vi "VI malcriado.vi"(8 "error in":errorcluster, 11 "This VI":refnum<vi>) -> ()   [LabVIEW 2024]
uses:
  <vilib>/Utility/miscctls.llb/LVRowAndColumnTypeDef.ctl
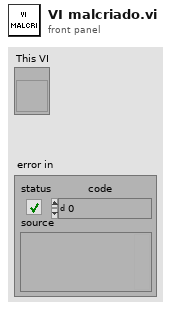
[diagram p1: front panel]
types:
  T1 = typedef "Pdash Style--cluster.ctl" = cluster{"Gris Obscuro Azul":u32, "Gris Medio Azul":u32, "Gris Claro Azul":u32, "Amarillo":u32, "Text color":u32, "Transparent":u32, "Fuente":string, "Text.Font:Size":u32}
  T2 = typedef "LVRowAndColumnTypeDef.ctl" = cluster{"Row":i32, "Column":i32}
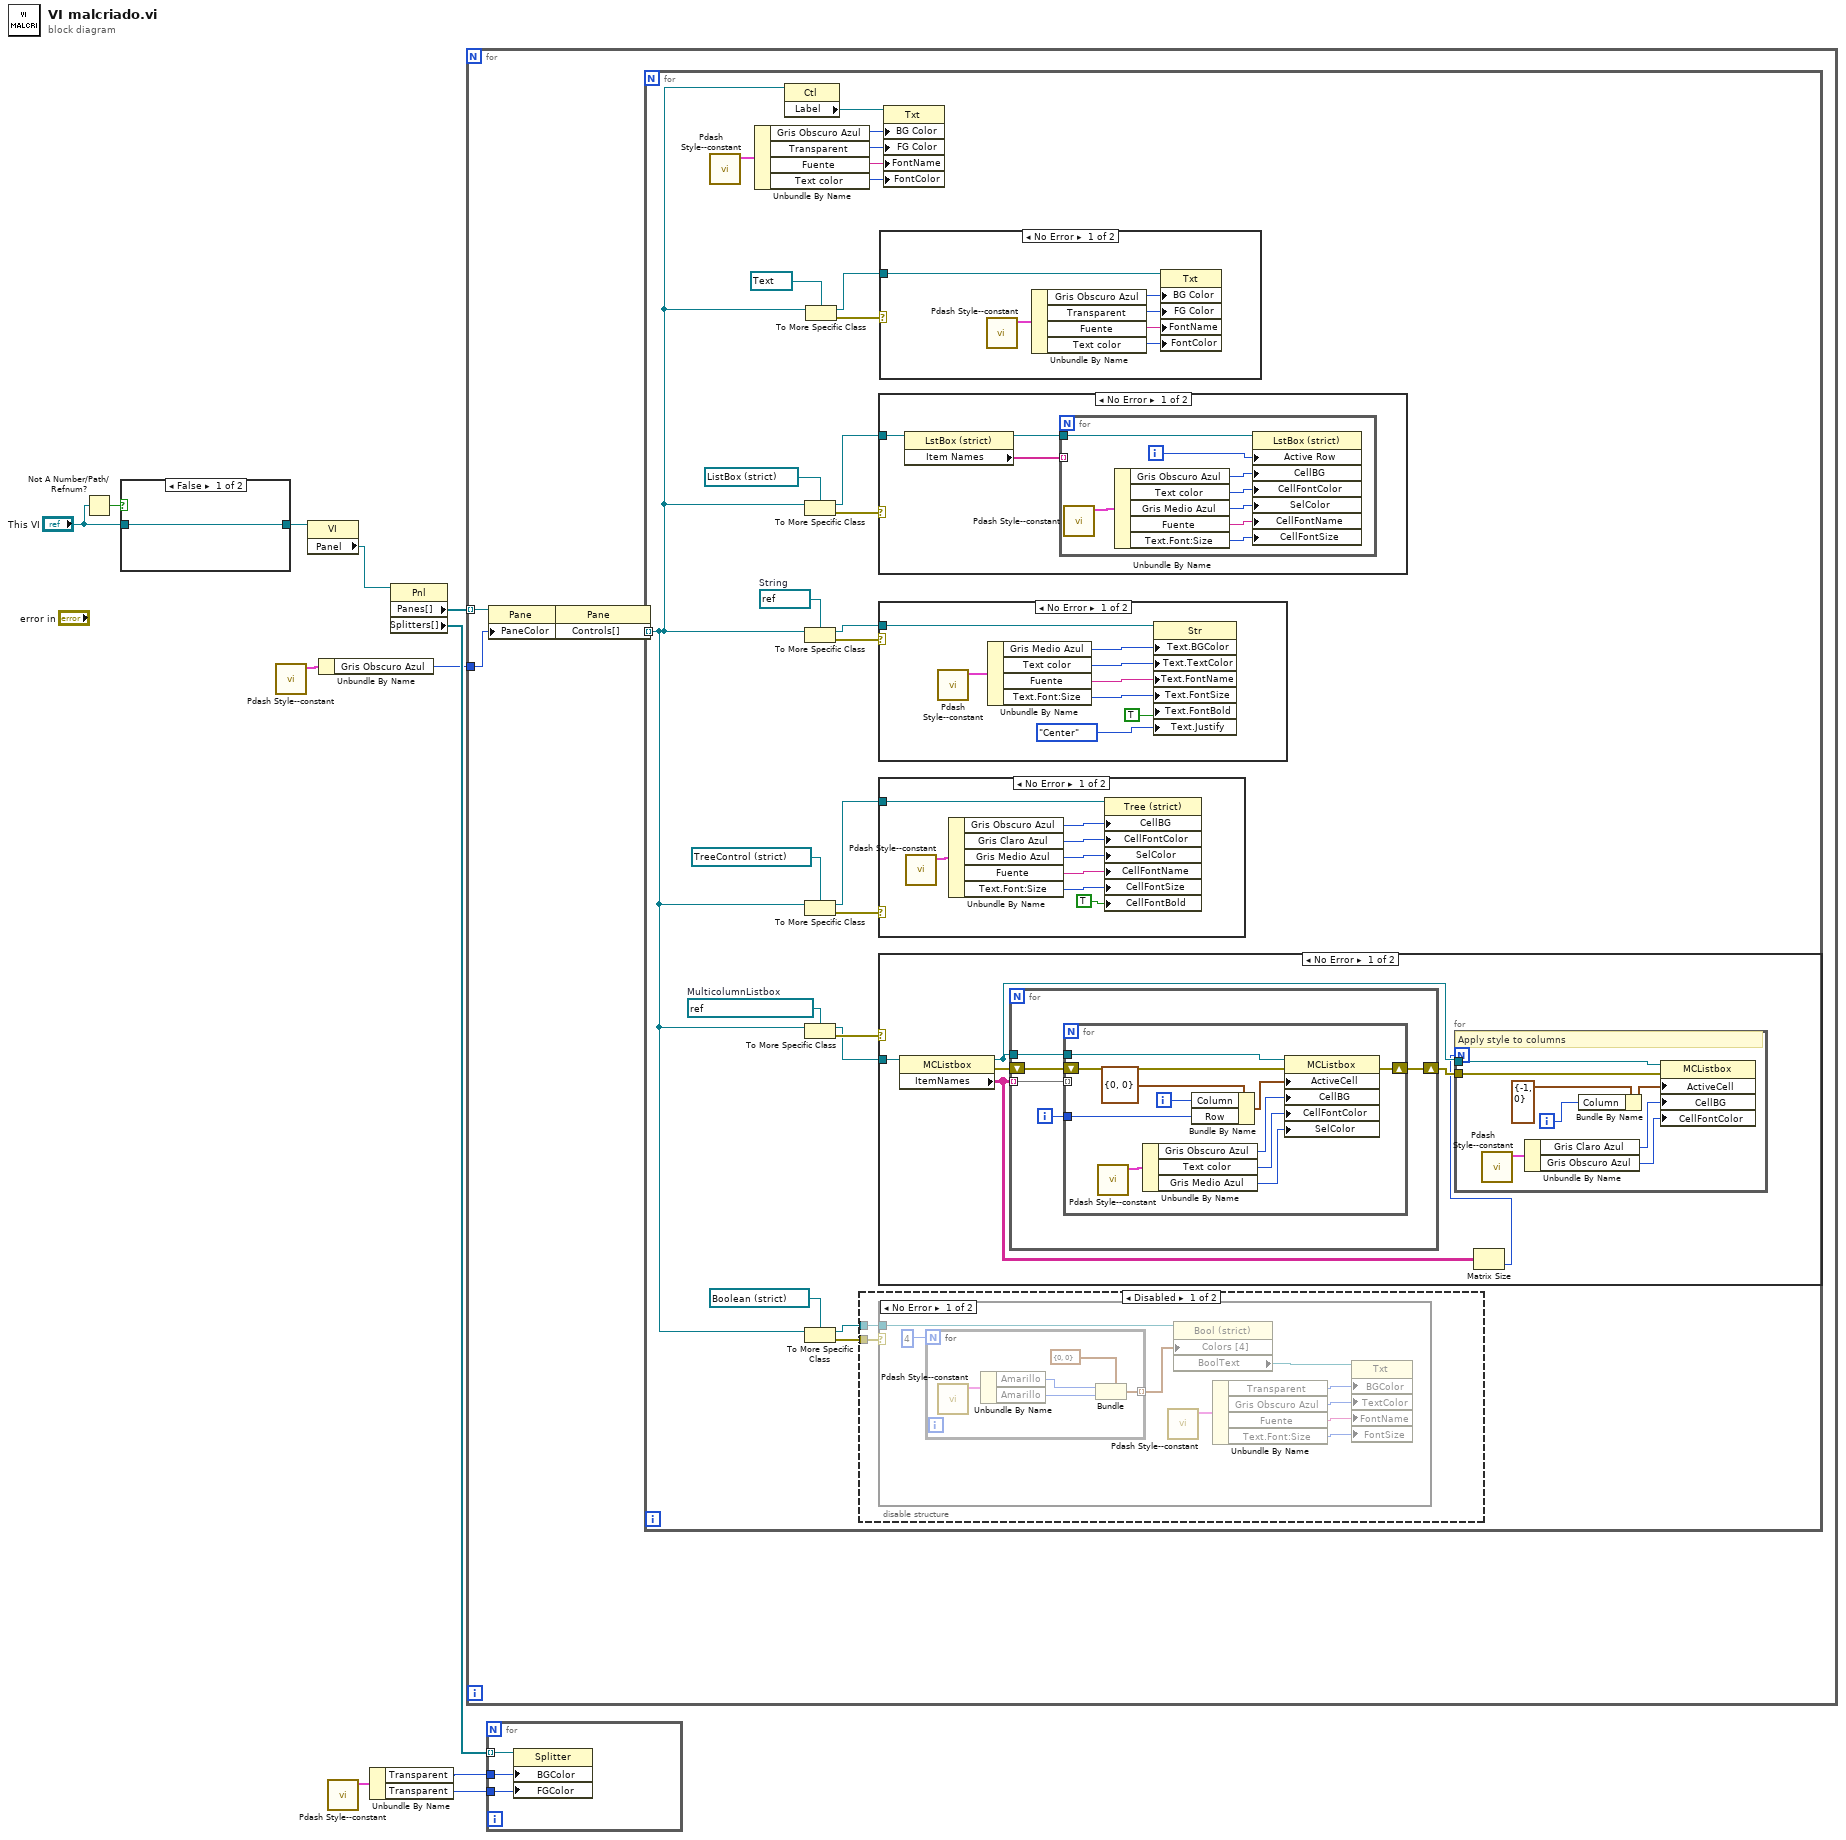
[diagram p0: block diagram]
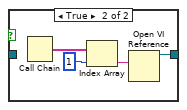
[diagram p9: hidden frame]
diagram:
  n1 = Not A Number/Path/Refnum?(number/path/refnum="This VI") -> (NaN/Path/Refnum?=w11:bool)
  n2 = case shown="False" w11 {
    tunnel: [w12 w13] -> w9
    tunnel: "This VI" -> [w12 _]
    frame False {
    }
    frame True {
      n3 = Call Chain() -> (call chain=w16:string[])
      n4 = Index Array(array=w16, index=1) -> (element=w14:string)
      n5 = Open VI Reference(vi path=w14) -> (vi reference=w13:refnum<vi>)  [unwired: 5 in, 1 out]
    }
  }
  n6 = call "Pdash Style--constant.vi"() -> ("Style"=w2:T1)  [unwired: 11 in]
  n7 = property class="VI"(reference=w9) -> ("Panel"=w8:refnum<vi>)  [unwired: 1 in, 2 out]
  n8 = Unbundle By Name(w2) -> ("Gris Obscuro Azul"=w1:u32)
  n9 = call "Pdash Style--constant.vi"() -> ("Style"=w5:T1)  [unwired: 11 in]
  n10 = Unbundle By Name(w5) -> ("Transparent"=w4:u32, "Transparent"=w3:u32)
  n11 = property class="Pnl"(reference=w8) -> ("Panes[]"=w7:refnum<vi>[], "Splitters[]"=w6:refnum<vi>[])  [unwired: 1 in, 2 out]
  n12 = for {
    tunnel: w7 -> [w20] mode=indexing
    tunnel: w1 -> [w17]
    n13 = property class="Pane"(reference=w20, "PaneColor"=w17) -> (reference out=w19:refnum<vi>)  [unwired: 1 in, 1 out]
    n14 = property class="Pane"(reference=w19) -> ("Controls[]"=w18:refnum<vi>[])  [unwired: 1 in, 2 out]
    n15 = for {
      tunnel: w18 -> [w22] mode=indexing
      w34 = refnum<vi> refnum  # String
      w35 = refnum<vi> refnum  # MulticolumnListbox
      n16 = call "Pdash Style--constant.vi"() -> ("Style"=w31:T1)  [unwired: 11 in]
      n17 = Unbundle By Name(w31) -> ("Gris Obscuro Azul"=w30:u32, "Transparent"=w27:u32, "Fuente"=w29:string, "Text color"=w28:u32)
      n18 = property class="Ctl"(reference=w22) -> ("Label"=w32:refnum<vi>)  [unwired: 1 in, 2 out]
      n19 = To More Specific Class(target class=refnum<vi> refnum ("Project history"), reference=w22) -> (specific class reference=w37:refnum<vi>, error out=w43:errorcluster)  [unwired: 1 in]
      n20 = To More Specific Class(target class=w34, reference=w22) -> (specific class reference=w33:refnum<vi>, error out=w41:errorcluster)  [unwired: 1 in]
      n21 = To More Specific Class(target class=refnum<vi> refnum ("Tree Control"), reference=w22) -> (specific class reference=w38:refnum<vi>, error out=w44:errorcluster)  [unwired: 1 in]
      n22 = To More Specific Class(target class=w35, reference=w22) -> (specific class reference=w36:refnum<vi>, error out=w42:errorcluster)  [unwired: 1 in]
      n23 = To More Specific Class(target class=refnum<vi> refnum ("Scan All"), reference=w22) -> (specific class reference=w39:refnum<vi>, error out=w45:errorcluster)  [unwired: 1 in]
      n24 = To More Specific Class(target class=refnum<vi> refnum ("Project history"), reference=w22) -> (specific class reference=w23:refnum<vi>, error out=w40:errorcluster)  [unwired: 1 in]
      n25 = disable-structure shown="Disabled" {
        disable-tunnel: w45 -> [w47 _]
        disable-tunnel: w39 -> [w46 _]
        frame Disabled {
          n26 = case shown="No Error" w47 {
            tunnel: w46 -> [w50 _]
            frame No Error {
              n27 = for {
                N: 4 -> [_]
                tunnel: [w60] -> w55 mode=indexing
                n28 = call "Pdash Style--constant.vi"() -> ("Style"=w59:T1)  [unwired: 11 in]
                n29 = Unbundle By Name(w59) -> ("Amarillo"=w57:u32, "Amarillo"=w58:u32)
                n30 = Bundle(cluster=cluster{u32, u32} {0, 0} ("Colors [4]"), w57, w58) -> (w60:cluster{u32, u32})
              }
              n31 = call "Pdash Style--constant.vi"() -> ("Style"=w53:T1)  [unwired: 11 in]
              n32 = property class="Bool (strict)"(reference=w50, "Colors [4]"=w55) -> ("BoolText"=w56:refnum<vi>)  [unwired: 1 in, 2 out]
              n33 = Unbundle By Name(w53) -> ("Transparent"=w52:u32, "Gris Obscuro Azul"=w51:u32, "Fuente"=w49:string, "Text.Font:Size"=w48:u32)
              n34 = property class="Txt"(reference=w56, "BGColor"=w52, "TextColor"=w51, "FontName"=w49, "FontSize"=w48) -> ()  [unwired: 1 in, 2 out]
            }
            frame Error {
            }
          }
        }
        frame Enabled {
        }
      }
      n35 = case shown="No Error" w43 {
        tunnel: w37 -> [w116 _]
        frame No Error {
          n36 = property class="LstBox (strict)"(reference=w116) -> (reference out=w115:refnum<vi>, "Item Names"=w114:string[])  [unwired: 1 in, 1 out]
          n37 = for {
            tunnel: w115 -> [w119]
            tunnel: w114 -> [_] mode=indexing
            i -> [w117]
            n38 = call "Pdash Style--constant.vi"() -> ("Style"=w124:T1)  [unwired: 11 in]
            n39 = Unbundle By Name(w124) -> ("Gris Obscuro Azul"=w118:u32, "Text color"=w123:u32, "Gris Medio Azul"=w122:u32, "Fuente"=w121:string, "Text.Font:Size"=w120:u32)
            n40 = property class="LstBox (strict)"(reference=w119, "Active Row"=w117, "CellBG"=w118, "CellFontColor"=w123, "SelColor"=w122, "CellFontName"=w121, "CellFontSize"=w120) -> ()  [unwired: 1 in, 2 out]
          }
        }
        frame Error {
        }
      }
      n41 = case shown="No Error" w41 {
        tunnel: w33 -> [w75 _]
        frame No Error {
          n42 = call "Pdash Style--constant.vi"() -> ("Style"=w74:T1)  [unwired: 11 in]
          n43 = Unbundle By Name(w74) -> ("Gris Medio Azul"=w73:u32, "Text color"=w72:u32, "Fuente"=w71:string, "Text.Font:Size"=w70:u32)
          n44 = property class="Str"(reference=w75, "Text.BGColor"=w73, "Text.TextColor"=w72, "Text.FontName"=w71, "Text.FontSize"=w70, "Text.FontBold"=TRUE ("Text.Font:Bold"), "Text.Justify"=enum16{"Left", "Center", "Right"}."Center" ("Text.Justification")) -> ()  [unwired: 1 in, 2 out]
        }
        frame Error {
        }
      }
      n45 = case shown="No Error" w44 {
        tunnel: w38 -> [w108 _]
        frame No Error {
          n46 = call "Pdash Style--constant.vi"() -> ("Style"=w113:T1)  [unwired: 11 in]
          n47 = Unbundle By Name(w113) -> ("Gris Obscuro Azul"=w112:u32, "Gris Claro Azul"=w111:u32, "Gris Medio Azul"=w110:u32, "Fuente"=w109:string, "Text.Font:Size"=w107:u32)
          n48 = property class="Tree (strict)"(reference=w108, "CellBG"=w112, "CellFontColor"=w111, "SelColor"=w110, "CellFontName"=w109, "CellFontSize"=w107, "CellFontBold"=TRUE ("Active Cell:Cell Font:Bold")) -> ()  [unwired: 1 in, 2 out]
        }
        frame Error {
        }
      }
      n49 = case shown="No Error" w42 {
        tunnel: w36 -> [w79 _]
        frame No Error {
          n50 = property class="MCListbox"(reference=w79) -> (reference out=w78:refnum<vi>, error out=w81:errorcluster, "ItemNames"=w77:string[][])  [unwired: 1 in]
          n51 = for {
            tunnel: w78 -> [w92]
            tunnel: w77 -> [w90] mode=indexing
            shift-right: [w93] -> w80
            shift-left: w81 -> [w94]
            i -> [w91]
            n52 = for {
              tunnel: w92 -> [w100]
              tunnel: w91 -> [w95]
              tunnel: w90 -> [_] mode=indexing
              shift-right: [w104] -> w93
              shift-left: w94 -> [w105]
              i -> [w96]
              n53 = call "Pdash Style--constant.vi"() -> ("Style"=w103:T1)  [unwired: 11 in]
              n54 = Unbundle By Name(w103) -> ("Gris Obscuro Azul"=w99:u32, "Text color"=w102:u32, "Gris Medio Azul"=w101:u32)
              n55 = Bundle By Name(cluster=T2 {"Row"=0, "Column"=0} ("Active Cell:Active Cell"), "Column"=w96, "Row"=w95) -> (w97:T2)
              n56 = property class="MCListbox"(reference=w100, error in=w105, "ActiveCell"=w97, "CellBG"=w99, "CellFontColor"=w102, "SelColor"=w101) -> (error out=w104:errorcluster)  [unwired: 1 out]
            }
          }
          n57 = Matrix Size(0:w77) -> (2:w76:i32)  [unwired: 1 out]
          n58 = for {
            N: w76 -> [_]
            tunnel: w80 -> [w89]
            tunnel: w78 -> [w88]
            i -> [w82]
            # "Apply style to columns"
            n59 = call "Pdash Style--constant.vi"() -> ("Style"=w86:T1)  [unwired: 11 in]
            n60 = Unbundle By Name(w86) -> ("Gris Claro Azul"=w85:u32, "Gris Obscuro Azul"=w84:u32)
            n61 = Bundle By Name(cluster=T2 {"Row"=-1, "Column"=0} ("Active Cell:Active Cell"), "Column"=w82) -> (w83:T2)
            n62 = property class="MCListbox"(reference=w88, error in=w89, "ActiveCell"=w83, "CellBG"=w85, "CellFontColor"=w84) -> ()  [unwired: 2 out]
          }
        }
        frame Error {
        }
      }
      n63 = case shown="No Error" w40 {
        tunnel: w23 -> [w62 _]
        frame No Error {
          n64 = call "Pdash Style--constant.vi"() -> ("Style"=w67:T1)  [unwired: 11 in]
          n65 = Unbundle By Name(w67) -> ("Gris Obscuro Azul"=w66:u32, "Transparent"=w63:u32, "Fuente"=w65:string, "Text color"=w64:u32)
          n66 = property class="Txt"(reference=w62, "BG Color"=w66, "FG Color"=w63, "FontName"=w65, "FontColor"=w64) -> ()  [unwired: 1 in, 2 out]
        }
        frame Error {
        }
      }
      n67 = property class="Txt"(reference=w32, "BG Color"=w30, "FG Color"=w27, "FontName"=w29, "FontColor"=w28) -> ()  [unwired: 1 in, 2 out]
    }
  }
  n68 = for {
    tunnel: w6 -> [w127] mode=indexing
    tunnel: w4 -> [w126]
    tunnel: w3 -> [w125]
    n69 = property class="Splitter"(reference=w127, "BGColor"=w126, "FGColor"=w125) -> ()  [unwired: 1 in, 2 out]
  }
